vi "Check Target LV Package Version.vi"(8 "Error In":errorcluster, 11 "Install LV Data":T1={"SSH Session"=refnum, "Status Log"="", "Detailed Log"="", "Credentials"={"Hostname or IP"="192.168.7.2", "Username"="root", "Password"=""}, "Target Info"={"OS Version"="", "CPU"="", "Systemd Version"="", "Internet Access"=FALSE, "Device Type"="", "LV Installed Ver"="", "LV Available Ver"="", "LV Upgrade Available"=FALSE, "Hostname"="", "NIC Info"=[]}, "Reboot Required?"=FALSE}) -> (0 "Error Out":errorcluster, 1 "Available Version":string, 2 "Installed Version":string, 3 "Install LV Data":T1={"SSH Session"=refnum, "Status Log"="", "Detailed Log"="", "Credentials"={"Hostname or IP"="192.168.7.2", "Username"="root", "Password"=""}, "Target Info"={"OS Version"="", "CPU"="", "Systemd Version"="", "Internet Access"=FALSE, "Device Type"="", "LV Installed Ver"="", "LV Available Ver"="", "LV Upgrade Available"=FALSE, "Hostname"="", "NIC Info"=[]}, "Reboot Required?"=FALSE}, 4 "Upgrade Available?":bool)   [LabVIEW 2020, in "LMH-LINX.lvlib"]
uses:
  LMH-LINX.lvlib
  Install LV Data.ctl
  Target Info.ctl
  NIC Info.ctl
  NIC Mode.ctl
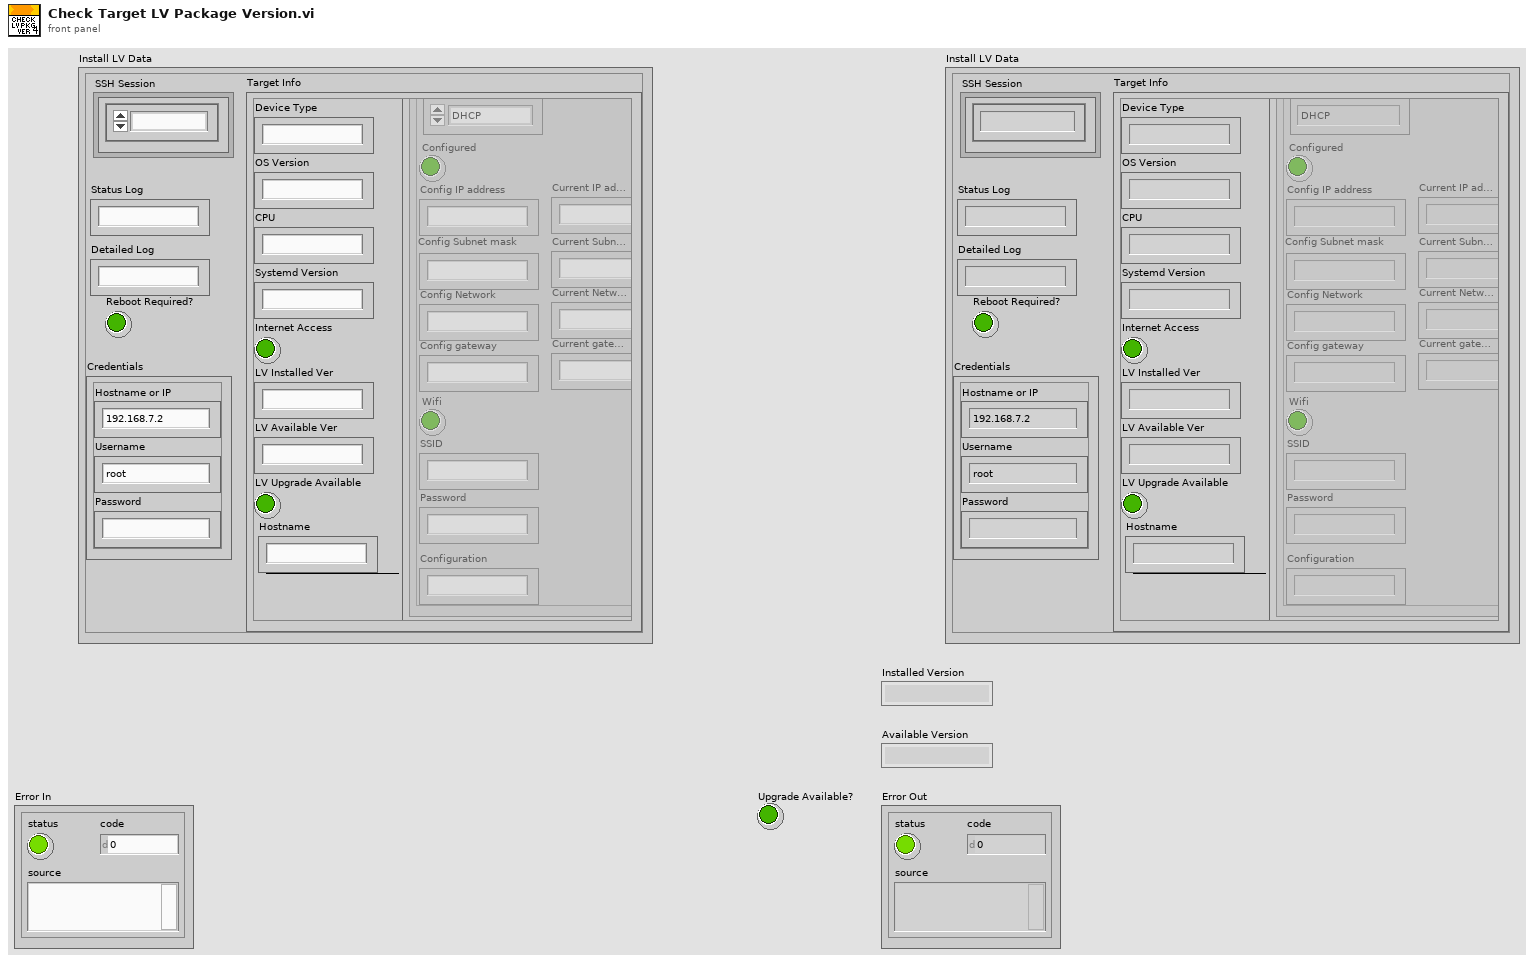
[diagram p1: front panel]
types:
  T1 = typedef "LMH-LINX.lvlib/Install LV Data.ctl" = cluster{"SSH Session":refnum<k1>, "Status Log":string, "Detailed Log":string, "Credentials":cluster{"Hostname or IP":string, "Username":string, "Password":string}, "Target Info":T2, "Reboot Required?":bool}
  T2 = typedef "LMH-LINX.lvlib/Target Info.ctl" = cluster{"OS Version":string, "CPU":string, "Systemd Version":string, "Internet Access":bool, "Device Type":string, "LV Installed Ver":string, "LV Available Ver":string, "LV Upgrade Available":bool, "Hostname":string, "NIC Info":T3[]}
  T3 = typedef "LMH-LINX.lvlib/NIC Info.ctl" = cluster{"Name":string, "NIC Mode":T4, "Configured":bool, "Config IP address":string, "Config Subnet mask":string, "Config Network":string, "Config gateway":string, "Wifi":bool, "SSID":string, "Password":string, "Configuration":string, "Current IP address":string, "Current Subnet mask":string, "Current gateway":string, "Current Network":string}
  T4 = typedef "LMH-LINX.lvlib/NIC Mode.ctl" = enum16{"DHCP", "Static", "Loopback"}
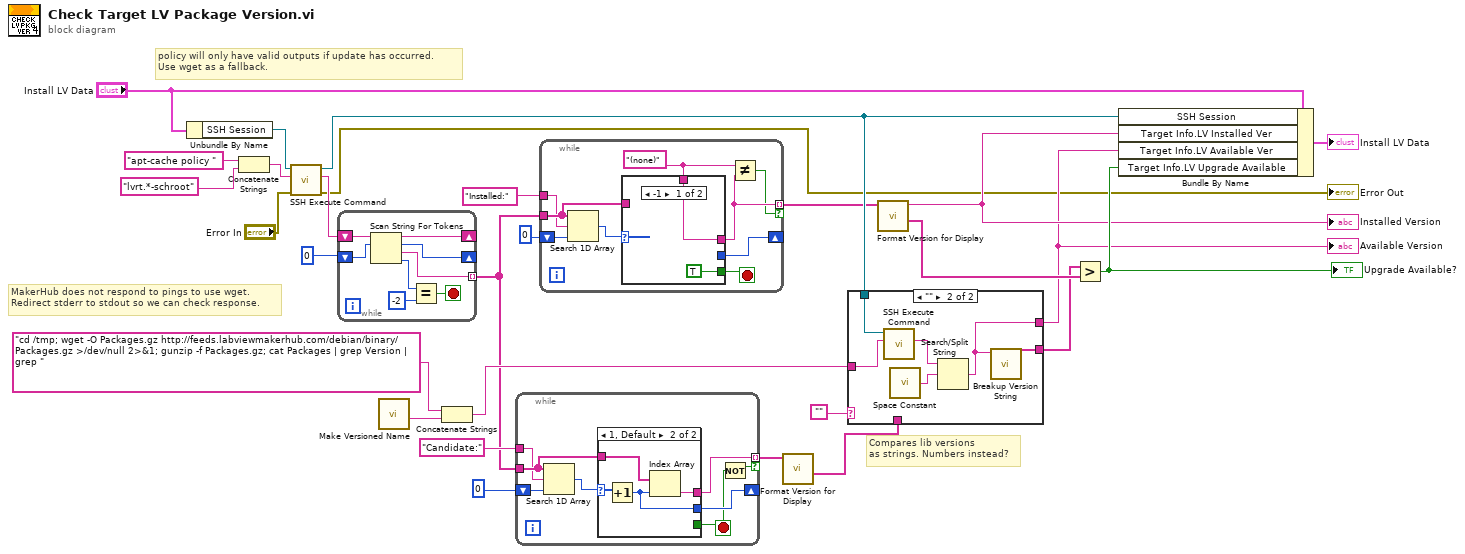
[diagram p0: block diagram]
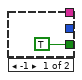
[diagram p2: hidden frame]
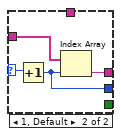
[diagram p3: hidden frame]
diagram:
  # "Compares lib versions\nas strings. Numbers instead?"
  # "policy will only have valid outputs if update has occurred.\nUse wget as a fallback."
  # "MakerHub does not respond to pings to use wget.\nRedirect stderr to stdout so we can check response."
  n1 = Unbundle By Name("Install LV Data") -> ("SSH Session"=w27:refnum<k1>)
  n2 = Concatenate Strings("apt-cache policy " ("Command"), "lvrt.*-schroot" ("Command")) -> (w20:string)
  n3 = call "SSH Execute Command.vi"("Error In"="Error In", "Command"=w20, "SSH Session"=w27) -> ("Error Out"=→"Error Out":errorcluster, "Std Out"=w23:string, "SSH Session"=w22:refnum<k1>)  [unwired: 6 in]
  n4 = while {
    shift-right: [w34] -> _
    shift-left: w23 -> [w36]
    shift-right: [w33] -> _
    shift-left: 0 -> [w35]
    tunnel: [w32] -> w11 mode=indexing
    stop <- w30 stop-if-true
    n5 = Scan String For Tokens(8:w35, 9:w36) -> (0:w29:i32, 1:w32:string, 2:w33:i32, 3:w34:string)  [unwired: 4 in]
    n6 = Equal?(x=w29, y=-2) -> (x = y?=w30:bool)
  }
  n7 = call "Make Versioned Name.vi"() -> ("LV Version"=w16:string)  [unwired: 10 in, 1 out]
  n8 = Concatenate Strings("cd /tmp; wget -O Packages.gz http://feeds.labviewmakerhub.com/debian/binary/Packages.gz >/dev/null 2>&1; gunzip -f Packages.gz; cat Packages | grep Version | grep " ("Command"), w16) -> (w17:string)
  n9 = while {
    tunnel: w11 -> [w43]
    tunnel: [w39] -> w7 mode=indexing if=w38
    shift-right: [w41] -> _
    shift-left: 0 -> [w42]
    tunnel: "Candidate:" ("element") -> [w40]
    stop <- w37 stop-if-true
    n10 = Search 1D Array(1D array=w43, element=w40, start index (0)=w42) -> (index of element=w44:i32)
    n11 = case shown="1, Default" w44 {
      selector: w44 -> [_ w49]
      tunnel: w43 -> [_ w48]
      tunnel: [_ w47] -> w39
      tunnel: [TRUE _] -> w37
      tunnel: [_ w46] -> w41
      frame -1 {
      }
      frame 1, Default {
        n12 = Increment(x=w49) -> (x+1=w46:i32)
        n13 = Index Array(array=w48, index=w46) -> (element=w47:string)
      }
    }
    n14 = Not(x=w37) -> (.not. x?=w38:bool)
  }
  n15 = while {
    tunnel: w11 -> [w57]
    tunnel: [w52] -> w9 mode=indexing if=w51
    shift-right: [w54] -> _
    shift-left: 0 -> [w56]
    tunnel: "Installed:" ("element") -> [w53]
    stop <- w55 stop-if-true
    w50 = "(none)" ("element")
    n16 = Search 1D Array(1D array=w57, element=w53, start index (0)=w56) -> (index of element=w58:i32)
    n17 = case shown="-1" w58 {
      selector: w58 -> [_ w64]
      tunnel: w57 -> [_ w63]
      tunnel: [w59 w62] -> w52
      tunnel: [TRUE _] -> w55
      tunnel: [_ w61] -> w54
      tunnel: w50 -> [w59 _]
      frame -1 {
      }
      frame 1, Default {
        n18 = Increment(x=w64) -> (x+1=w61:i32)
        n19 = Index Array(array=w63, index=w61) -> (element=w62:string)
      }
    }
    n20 = Not Equal?(x=w50, y=w52) -> (x != y?=w51:bool)
  }
  n21 = call "Format Version for Display.vi"("Strings"=w7) -> ("Latest Vers"=w5:string[])  [unwired: 8 in, 2 out]
  n22 = case shown="\"\"" "" {
    selector: "" -> [w66 _]
    tunnel: w22 -> [_ w71]
    tunnel: [w66 w67] -> w3
    tunnel: w17 -> [_ w69]
    tunnel: w5 -> [w65 _]
    tunnel: [w65 w68] -> w4
    frame Default {
    }
    frame "" {
      n23 = call "SSH Execute Command.vi"("Command"=w69, "SSH Session"=w71) -> ("Std Out"=w70:string)  [unwired: 7 in, 2 out]
      n24 = call <vilib>:"Space Constant.vi"() -> ("String"=w72:string)
      n25 = Search/Split String(string=w70, search string/char (-)=w72) -> (match + rest of string=w67:string)  [unwired: 1 in, 2 out]
      n26 = call "Breakup Version String.vi"("Vers String"=w67) -> ("Substrings"=w68:string[])  [unwired: 10 in]
    }
  }
  "Available Version" <- w3
  n27 = call "Format Version for Display.vi"("Strings"=w9) -> ("Latest Vers"=w6:string[], "String"=w8:string)  [unwired: 8 in, 1 out]
  "Installed Version" <- w8
  n28 = Greater?(x=w4, y=w6) -> (0:w24:bool)
  "Upgrade Available?" <- w24
  n29 = Bundle By Name(cluster="Install LV Data", "SSH Session"=w22, "Target Info.LV Installed Ver"=w8, "Target Info.LV Available Ver"=w3, "Target Info.LV Upgrade Available"=w24) -> (→"Install LV Data":T1)
